vi "Test SlideBackgroundGradient.vi"() -> ()   [LabVIEW 2015, in "SlideBackgroundGradient.lvclass"]
doc: "<b> </b> <b> </b>\n©2016 Q Software Innovations, LLC (QSI)\nwritten by Quentin Alldredge\nproduced in LabVIEW 2015\n\nsupport@qsoftwareinnovations.com\nwww.qsoftwareinnovations.com\n\nAll rights reserved.\n\nRedistribution and use in source and binary forms, with or without modification, are permitted provided that the following conditions are met:\n\n * Redistributions of source code must retain the above copyright notice, this list of conditions and the following disclaimer.\n * Redistributions in binary form must reproduce the above copyright notice, this list of conditions and the following disclaimer in the documentation and/or other materials provided with the distribution.\n * Neither the name of Q Software Innovations, LLC. nor the names of its contributors may be used to endorse or promote products derived from this software without specific prior written permission.\n\nTHIS SOFTWARE IS PROVIDED BY THE COPYRIGHT HOLDERS AND CONTRIBUTORS \"AS IS\" AND ANY EXPRESS OR IMPLIED WARRANTIES, INCLUDING, BUT NOT LIMITED TO, THE IMPLIED WARRANTIES OF MERCHANTABILITY AND FITNESS FOR A PARTICULAR PURPOSE ARE DISCLAIMED. IN NO EVENT SHALL THE COPYRIGHT OWNER OR CONTRIBUTORS BE LIABLE FOR ANY DIRECT, INDIRECT, INCIDENTAL, SPECIAL, EXEMPLARY, OR CONSEQUENTIAL DAMAGES (INCLUDING, BUT NOT LIMITED TO, PROCUREMENT OF SUBSTITUTE GOODS OR SERVICES; LOSS OF USE, DATA, OR PROFITS; OR BUSINESS INTERRUPTION) HOWEVER CAUSED AND ON ANY THEORY OF LIABILITY, WHETHER IN CONTRACT, STRICT LIABILITY, OR TORT (INCLUDING NEGLIGENCE OR OTHERWISE) ARISING IN ANY WAY OUT OF THE USE OF THIS SOFTWARE, EVEN IF ADVISED OF THE POSSIBILITY OF SUCH DAMAGE."
uses:
  SlideBackgroundGradient.lvclass
  Write StartColor.vi
  Write EndColor.vi
panel:
  in  "Slide":dbl(slide) scale=-10.0..10.0
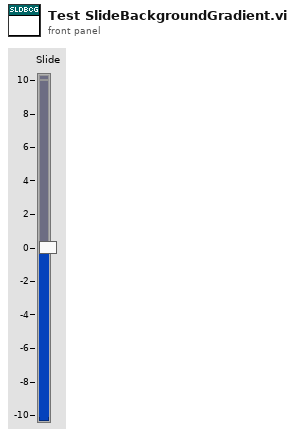
[diagram p1: front panel]
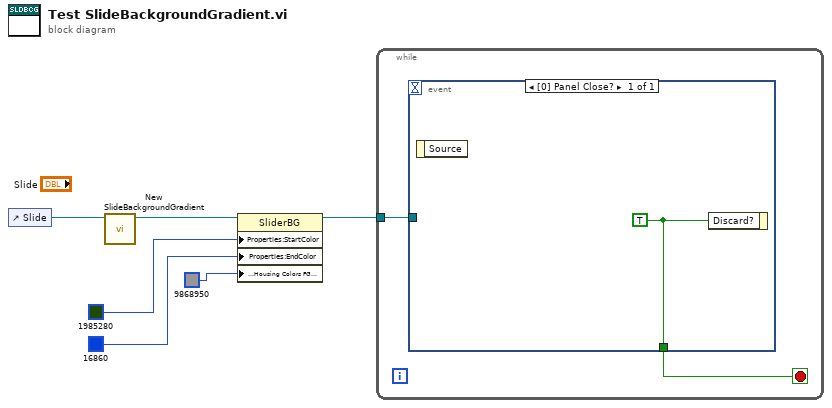
[diagram p0: block diagram]
diagram:
  n1 = control-ref of="Slide"() -> (w2:refnum<vi>)
  n2 = call "New SlideBackgroundGradient.vi"("Reference"=w2) -> ("SlideBackgroundGradient out"=w6:refnum<class "SlideBackgroundGradient.lvclass">)  [unwired: 9 in, 1 out]
  n3 = property class="SliderBG"(reference=w6, "Properties:StartColor"=u32 1985280, "Properties:EndColor"=u32 16860, "Properties:Housing Colors FG Color"=u32 9868950) -> (reference out=w5:refnum<class "SlideBackgroundGradient.lvclass">)  [unwired: 1 in, 1 out]
  n4 = while {
    tunnel: w5 -> [w7]
    stop <- w8 stop-if-true
    n5 = event shown="[0] Panel Close?" {
      selector: _ -> [_]
      dyn-events: _ -> [_]
      timeout: _ -> [_]
      tunnel: [w9] -> w8
      tunnel: w7 -> [_]
      event Panel Close? {
        w9 = TRUE
        n6 = event-data() -> ()  [unwired: 1 in, 1 out]
        n7 = event-data("Discard?"=w9) -> ()  [unwired: 1 in, 1 out]
      }
    }
  }
